vi "CRYGet StepVIFileRef.vi"(7 "Category":string, 10 "Step Name":string) -> (1 "Step Name Replace VI ref":refnum<vi>, 2 "Step Run VI ref":refnum<vi>, 3 "Step Edit VI ref":refnum<vi>)   [LabVIEW 2013]
uses:
  CRYMainGlobal.vi
  CRYSystem/Program/CRYRef nums global.vi
panel:
  in  "type Name Replace VI":refnum<vi>
  in  "type specifier":refnum<vi>
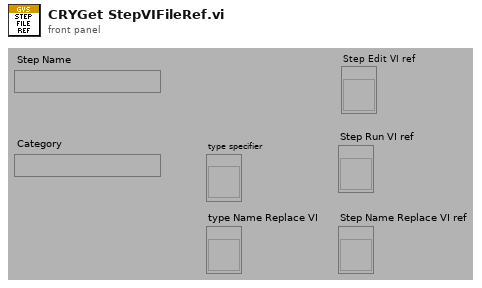
[diagram p1: front panel]
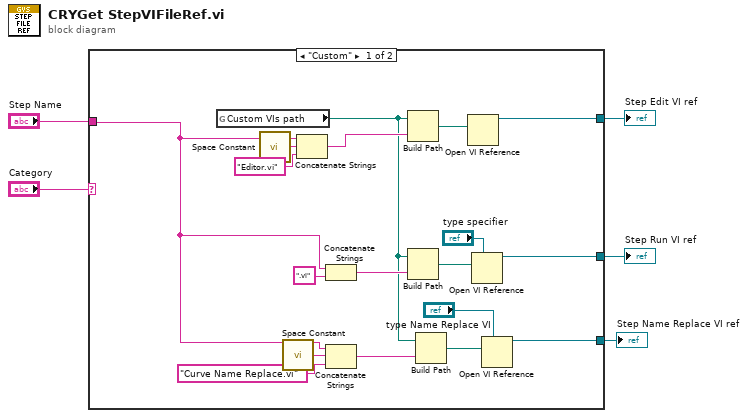
[diagram p0: block diagram]
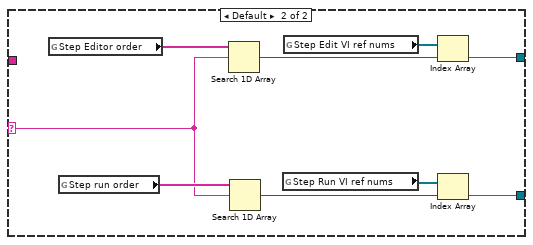
[diagram p2: hidden frame]
diagram:
  n1 = case shown="\"Custom\"" "Category" {
    selector: "Category" -> [_ w24]
    tunnel: [w16 w28] -> w5
    tunnel: [w15 w25] -> w2
    tunnel: "Step Name" -> [w9 _]
    tunnel: [w13 _] -> w1
    frame "Custom" {
      n2 = global read "CRYMainGlobal.vi" "Custom VIs path"() -> (w8:path)
      n3 = call <vilib>:"Space Constant.vi"() -> ("String"=w20:string)
      n4 = call <vilib>:"Space Constant.vi"() -> ("String"=w10:string)
      n5 = Concatenate Strings(w9, w20, "Editor.vi" ("string")) -> (w19:string)
      n6 = Concatenate Strings(w9, ".vi" ("string")) -> (w23:string)
      n7 = Concatenate Strings(w9, w10, "Curve Name Replace.vi" ("string")) -> (w11:string)
      n8 = Build Path(base path=w8, name or relative path=w19) -> (appended path=w18:path)
      n9 = Build Path(base path=w8, name or relative path=w23) -> (appended path=w17:path)
      n10 = Build Path(base path=w8, name or relative path=w11) -> (appended path=w6:path)
      n11 = Open VI Reference(vi path=w18) -> (vi reference=w16:refnum<vi>)  [unwired: 5 in, 1 out]
      n12 = Open VI Reference(type specifier VI Refnum (for type only)="type specifier", vi path=w17) -> (vi reference=w15:refnum<vi>)  [unwired: 4 in, 1 out]
      n13 = Open VI Reference(type specifier VI Refnum (for type only)="type Name Replace VI", vi path=w6) -> (vi reference=w13:refnum<vi>)  [unwired: 4 in, 1 out]
    }
    frame Default {
      n14 = global read "CRYMainGlobal.vi" "Step Editor order"() -> (w27:string[])
      n15 = global read "CRYMainGlobal.vi" "Step run order"() -> (w26:string[])
      n16 = Search 1D Array(1D array=w27, element=w24) -> (index of element=w32:i32)  [unwired: 1 in]
      n17 = Search 1D Array(1D array=w26, element=w24) -> (index of element=w29:i32)  [unwired: 1 in]
      n18 = global read "CRYRef nums global.vi" "Step Run VI ref nums"() -> (w30:refnum<vi>[])
      n19 = global read "CRYRef nums global.vi" "Step Edit VI ref nums"() -> (w31:refnum<vi>[])
      n20 = Index Array(array=w31, index=w32) -> (element=w28:refnum<vi>)
      n21 = Index Array(array=w30, index=w29) -> (element=w25:refnum<vi>)
    }
  }
  "Step Run VI ref" <- w2
  "Step Edit VI ref" <- w5
  "Step Name Replace VI ref" <- w1
